vi "send set to epics.vi"(7 "Param Cluster":T1, 8 "error in":errorcluster, 9 "Value":variant, 10 "select":string, 11 "IOC Selected":string="hama_l9421_02_1") -> (0 "error out":errorcluster, 2 "Status":bool)   [LabVIEW 2022 SP3]
uses:
  pectus/control/Param Epics Cluster.ctl
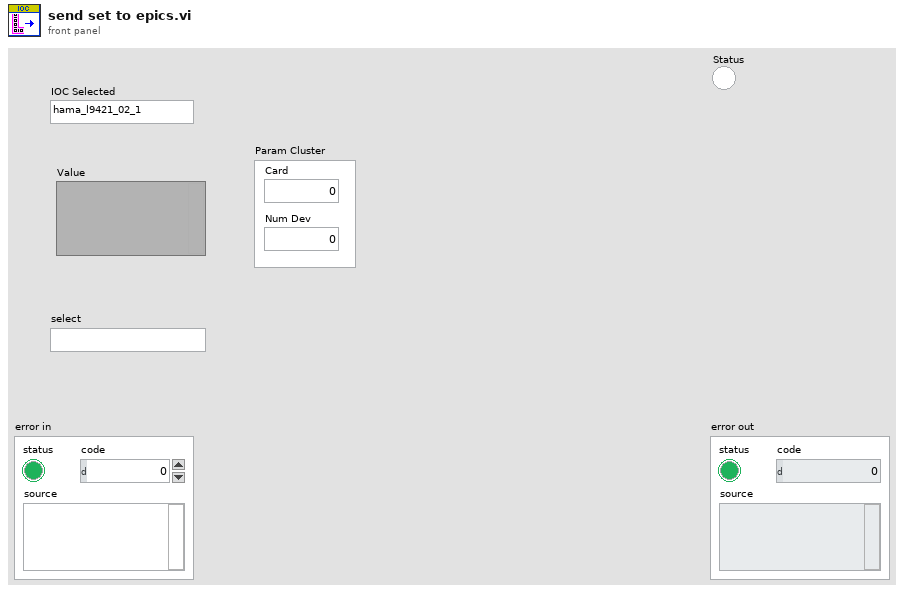
[diagram p1: front panel]
types:
  T1 = typedef "Param Epics Cluster.ctl" = cluster{"Card":u16, "Num Dev":u16}
  T2 = typedef "ca cluster.ctl" = cluster{"record":string, "prefix":string, "CA":string}
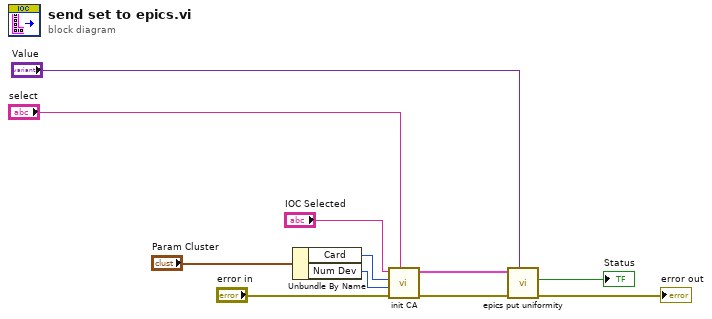
[diagram p0: block diagram]
diagram:
  n1 = Unbundle By Name("Param Cluster") -> ("Card"=w10:u16, "Num Dev"=w11:u16)
  n2 = call "init CA.vi"("Command"="select", "error in"="error in", "Device"=w11, "Card"=w10, "IOC"="IOC Selected") -> ("error out"=w6:errorcluster, "CA out"=w9:T2)  [unwired: 5 in]
  n3 = call "epics put uniformity.vi"("Value In"="Value", "error in"=w6, "CA in"=w9) -> ("error out"=→"error out":errorcluster, "Status"=→"Status":bool)  [unwired: 7 in]
